vi "subVI_CONEX_connectToStaticServerAndOpenCONEX-CCdevice.vi"(8 "Error IN":errorcluster, 9 "Connected devices":string[](array[string])=["COM3", "COM4 Newport CONEX-CC USB Serial Port (A6U3EQRMA\\0000)", "COM5 Newport CONEX-CC USB Serial Port (A6U3EQRMA\\0000)"], 10 "Controller Addresses":i32[](array[numeric])=[1, 1, 1], 11 "CONEX Client Lib Ref":refnum<k24>) -> (0 "error out":errorcluster caption="Error OUT", 1 "Addresses out":i32[](array[numeric]), 2 "Device Keys Out":string[](array[string]), 3 "CONEX Client Refs out":refnum<k24>[](array[refnum]), 4 "Info strings":string[](array[string]), 5 "IsOpened?":bool[](array[boolean]))   [LabVIEW 2010]
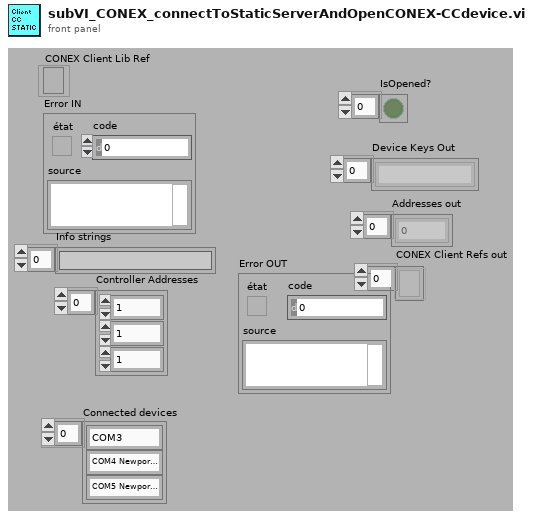
[diagram p1: front panel]
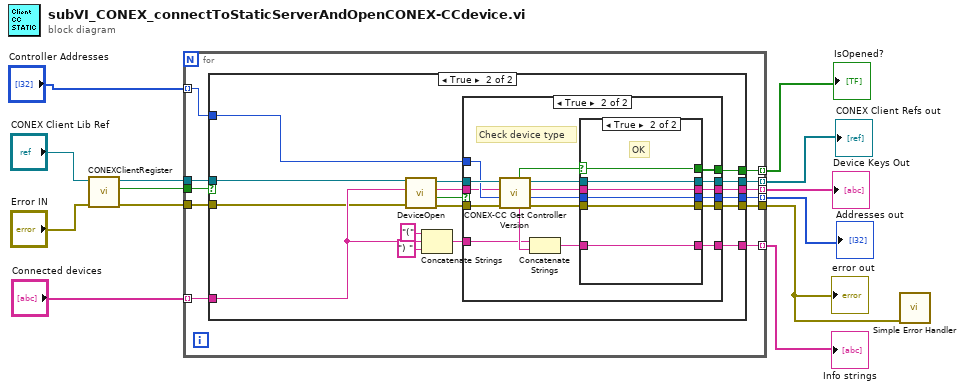
[diagram p0: block diagram]
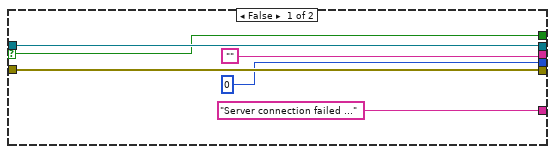
[diagram p2: hidden frame]
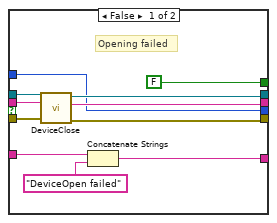
[diagram p3: hidden frame]
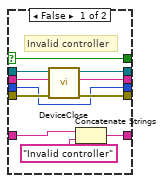
[diagram p4: hidden frame]
diagram:
  n1 = call <userlib>:"CONEXClientRegister.vi"("Error IN"="Error IN", "CONEX Client Lib Ref"="CONEX Client Lib Ref") -> ("Error OUT"=w11:errorcluster, "Connect?"=w12:bool, "CONEX Client Ref"=w13:refnum<k24>)  [unwired: 7 out]
  n2 = for {
    tunnel: w13 -> [w24]
    tunnel: w12 -> [w23]
    tunnel: w11 -> [w22]
    tunnel: [w21] -> w4 mode=indexing
    tunnel: [w20] -> w7 mode=indexing
    tunnel: [w19] -> w3 mode=indexing
    tunnel: [w18] -> w6 mode=indexing
    tunnel: [w17] -> w5 mode=indexing
    tunnel: [w16] -> w1
    tunnel: "Connected devices" -> [w15] mode=indexing
    tunnel: "Controller Addresses" -> [w14] mode=indexing
    n3 = case shown="True" w23 {
      selector: w23 -> [w25 _]
      tunnel: w24 -> [w29 w32]
      tunnel: w22 -> [w28 w31]
      tunnel: [w25 w40] -> w20
      tunnel: [w29 w39] -> w19
      tunnel: ["" w38] -> w18
      tunnel: [0 ("Address OUT") w37] -> w17
      tunnel: [w28 w36] -> w16
      tunnel: ["Server connection failed ..." w35] -> w21
      tunnel: w15 -> [_ w33]
      tunnel: w14 -> [_ w34]
      frame False {
      }
      frame True {
        n4 = call <userlib>:"DeviceOpen.vi"("Error IN"=w31, "deviceKey IN"=w33, "CONEX Client Ref IN"=w32) -> ("Error OUT"=w44:errorcluster, "DeviceOpen"=w47:bool, "deviceKey OUT"=w45:string, "CONEX Client Ref OUT"=w46:refnum<k24>)  [unwired: 5 out]
        n5 = Concatenate Strings("(" ("chaîne"), w33, ") " ("chaîne")) -> (w41:string)
        n6 = case shown="True" w47 {
          tunnel: w46 -> [w58 w76]
          tunnel: w45 -> [w56 w72]
          tunnel: w44 -> [w57 w75]
          tunnel: w34 -> [w52 w74]
          tunnel: [FALSE ("IsConexCC?") w65] -> w40
          tunnel: [w55 w64] -> w39
          tunnel: [w54 w63] -> w38
          tunnel: [w52 w61] -> w37
          tunnel: [w53 w62] -> w36
          tunnel: w41 -> [w49 w71]
          tunnel: [w48 w59] -> w35
          frame False {
            # "Opening failed"
            n7 = call <userlib>:"DeviceClose.vi"("Error IN"=w57, "deviceKey IN"=w56, "CONEX Client Ref IN"=w58) -> ("Error OUT"=w53:errorcluster, "deviceKey OUT"=w54:string, "CONEX Client Ref OUT"=w55:refnum<k24>)  [unwired: 6 out]
            n8 = Concatenate Strings(w49, "DeviceOpen failed" ("Title")) -> (w48:string)
          }
          frame True {
            # "Check device type"
            n9 = call <userlib>:"CONEX-CC Get Controller Version.vi"("CONEX Client Ref IN"=w76, "deviceKey IN"=w72, "Address IN"=w74, "Error IN"=w75) -> ("IsConexCC?"=w70:bool, "Controller Version"=w73:string, "CONEX Client Ref OUT"=w69:refnum<k24>, "deviceKey OUT"=w68:string, "Address OUT"=w67:i32, "Error OUT"=w66:errorcluster)
            n10 = Concatenate Strings(w71, w73) -> (w60:string)
            n11 = case shown="True" w70 {
              selector: w70 -> [w84 w93]
              tunnel: w69 -> [w87 w92]
              tunnel: w68 -> [w86 w91]
              tunnel: w67 -> [w80 w89]
              tunnel: w66 -> [w85 w90]
              tunnel: [w84 w93] -> w65
              tunnel: [w83 w92] -> w64
              tunnel: [w82 w91] -> w63
              tunnel: [w81 w90] -> w62
              tunnel: [w80 w89] -> w61
              tunnel: w60 -> [w77 w88]
              tunnel: [w79 w88] -> w59
              frame False {
                # "Invalid controller"
                n12 = call <userlib>:"DeviceClose.vi"("Error IN"=w85, "deviceKey IN"=w86, "CONEX Client Ref IN"=w87) -> ("Error OUT"=w81:errorcluster, "deviceKey OUT"=w82:string, "CONEX Client Ref OUT"=w83:refnum<k24>)  [unwired: 6 out]
                n13 = Concatenate Strings(w77, "Invalid controller") -> (w79:string)
              }
              frame True {
                # "OK"
              }
            }
          }
        }
      }
    }
  }
  "error out" <- w1
  "IsOpened?" <- w7
  "Device Keys Out" <- w6
  "Addresses out" <- w5
  "Info strings" <- w4
  "CONEX Client Refs out" <- w3
  n14 = call <vilib>:"Simple Error Handler.vi"("error in (no error)"=w1) -> ()  [unwired: 4 in, 5 out]
